vi "Read ProductInfo.vi"(8 "error in (no error)":errorcluster, 11 "GeneralCar in":refnum<class "GeneralCar.lvclass">) -> (0 "error out":errorcluster, 2 "ProductInfo":string, 3 "GeneralCar out":refnum<class "GeneralCar.lvclass">)   [LabVIEW 2021, in "GeneralCar.lvclass"]
uses:
  GeneralCar.lvclass
  GeneralCar.lvclass/GeneralCar.ctl
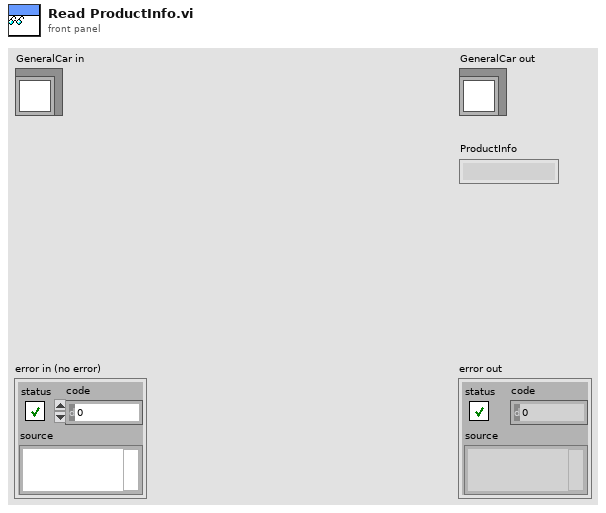
[diagram p1: front panel]
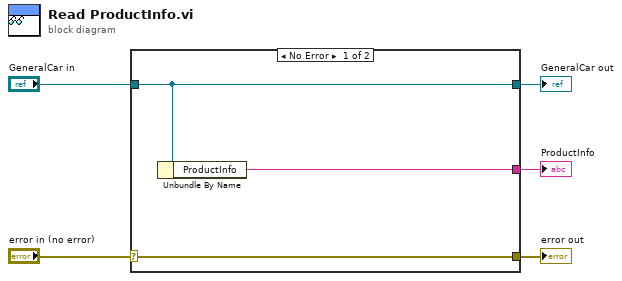
[diagram p0: block diagram]
diagram:
  n1 = case shown="No Error" "error in (no error)" {
    selector: "error in (no error)" -> [w8 w9]
    tunnel: [w8 w9] -> w4
    tunnel: [w7 w10] -> w2
    tunnel: "GeneralCar in" -> [w7 w10]
    tunnel: [w6 _] -> w1
    frame No Error {
      n2 = Unbundle By Name(w7) -> ("ProductInfo"=w6:string)
    }
    frame Error {
    }
  }
  "error out" <- w4
  "GeneralCar out" <- w2
  "ProductInfo" <- w1
